vi "binary to grey and viseversa.vi"() -> ()   [LabVIEW 2013]
panel:
  out "Boolean 7":bool
  out "Boolean 6":bool
  out "Boolean 5":bool
  out "Boolean 4":bool
  in  "Boolean 3":bool
  in  "Boolean 2":bool
  in  "Boolean":bool
  in  "Boolean":bool
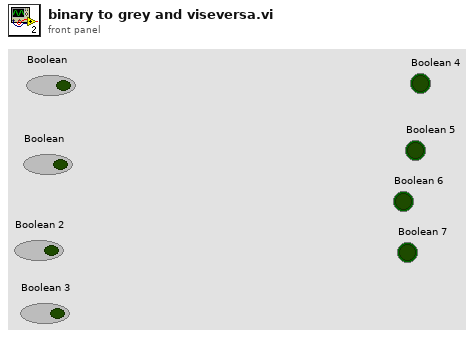
[diagram p1: front panel]
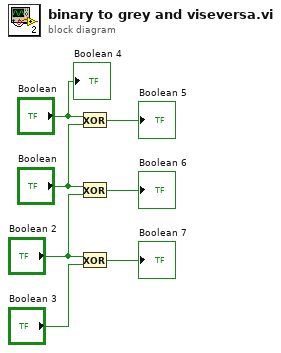
[diagram p0: block diagram]
diagram:
  n1 = Exclusive Or(1:"Boolean", 2:"Boolean") -> (0:→"Boolean 5":bool)
  n2 = Exclusive Or(1:"Boolean 2", 2:"Boolean") -> (0:→"Boolean 6":bool)
  n3 = Exclusive Or(1:"Boolean 3", 2:"Boolean 2") -> (0:→"Boolean 7":bool)
  "Boolean 4" <- "Boolean"
